vi "MathFunction.vi"(8 "error in (no error)":errorcluster, 9 "y":dbl, 10 "x":dbl, 11 "Add in":refnum<class "Add.lvclass">) -> (0 "error out":errorcluster, 2 "f(x,y)":dbl, 3 "Add out":refnum<class "Add.lvclass">)   [LabVIEW 2019, in "lv-classprovidershell-example.lvlib" / "Add.lvclass"]
uses:
  Add.lvclass
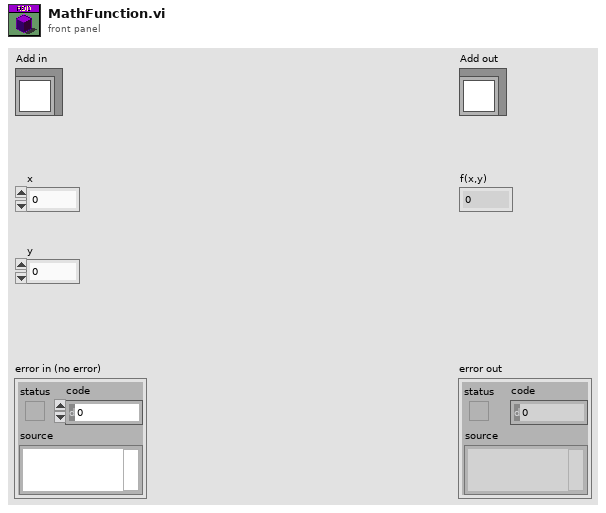
[diagram p1: front panel]
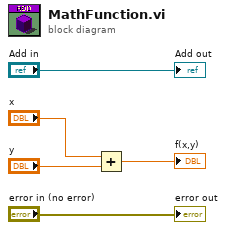
[diagram p0: block diagram]
diagram:
  n1 = Add(x="x", y="y") -> (x+y=→"f(x,y)":dbl)
  "error out" <- "error in (no error)"
  "Add out" <- "Add in"
